vi "TODO Run query.vi"(0 "Client.lvclass in":refnum<class "Client.lvclass">, 5 "Database name":string, 7 "Query":string, 9 "Precision":T1=enum."Nanoseconds", 11 "error in (no error)":errorcluster) -> (4 "Client.lvclass out":refnum<class "Client.lvclass">, 6 "JSON data":string, 15 "error out":errorcluster)   [LabVIEW 2018, in "InfluxDB Client.lvlib" / "Client.lvclass"]
doc: "Runs a query on a specific database and returns the result as JSON data."
uses:
  Client.lvclass
  Controls/Precision.ctl
  Client.lvclass/Client.ctl
  <vilib>/httpClient/LabVIEWHTTPClient.lvlib
  InfluxDB Client.lvlib
panel:
  out "Status":string
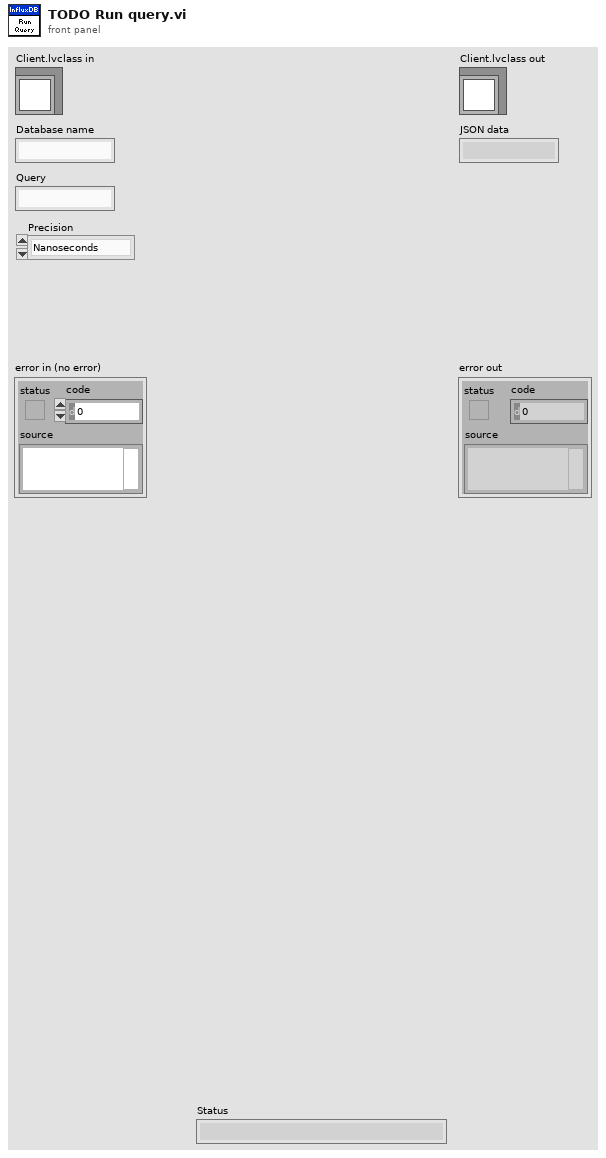
[diagram p1: front panel]
types:
  T1 = typedef "InfluxDB Client.lvlib/Precision.ctl" = enum16{"Seconds", "Milliseconds", "Nanoseconds"}
  T2 = typedef "LabVIEWHTTPClient.lvlib/ClientHandle.ctl" = refnum<k1>
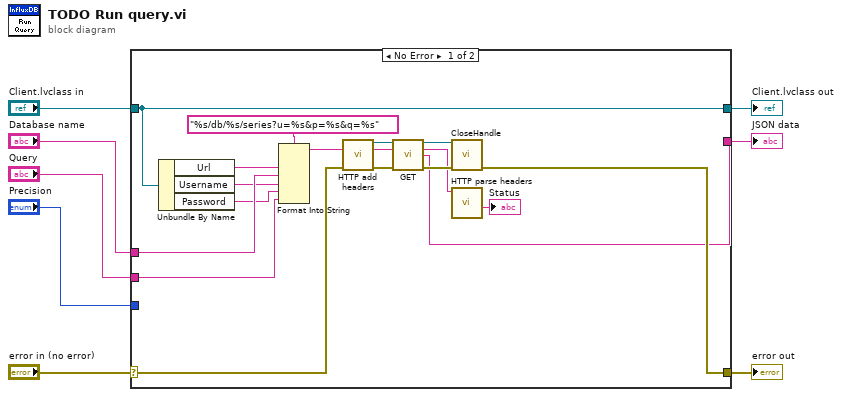
[diagram p0: block diagram]
diagram:
  n1 = case shown="No Error" "error in (no error)" {
    selector: "error in (no error)" -> [w11 w27]
    tunnel: [w19 w27] -> w7
    tunnel: [w25 w26] -> w5
    tunnel: "Client.lvclass in" -> [w25 w26]
    tunnel: [w12 _] -> w2
    tunnel: "Database name" -> [w16 _]
    tunnel: "Query" -> [w13 _]
    tunnel: "Precision" -> [_ _]
    frame No Error {
      n2 = Unbundle By Name(w25) -> ("Url"=w23:string, "Username"=w15:string, "Password"=w14:string)
      n3 = Format Into String(format string="%s/db/%s/series?u=%s&p=%s&q=%s" ("url"), w23, w16, w15, w14, w13) -> (resulting string=w20:string)  [unwired: 2 in, 1 out]
      n4 = call "HTTP add headers.vi"("error in (no error)"=w11) -> ("client handle out"=w10:T2, "error out"=w9:errorcluster)  [unwired: 13 in]
      n5 = call <vilib>:"GET.vi"("client handle"=w10, "url"=w20, "error in (no error)"=w9) -> ("client handle out"=w22:T2, "headers"=w18:string, "body"=w12:string, "error out"=w21:errorcluster)  [unwired: 9 in]
      n6 = call <vilib>:"CloseHandle.vi"("client handle"=w22, "error in (no error)"=w21) -> ("error out"=w19:errorcluster)  [unwired: 13 in]
      n7 = call "HTTP parse headers.vi"("HTTP headers"=w18) -> ("Status"=→"Status":string)  [unwired: 7 in, 3 out]
    }
    frame Error {
    }
  }
  "error out" <- w7
  "Client.lvclass out" <- w5
  "JSON data" <- w2
